vi "encryptSign.vi"(0 "HGF_GPG":refnum<class "HGF_GPG.lvclass">, 1 "options file":path, 2 "keyringfile":path, 3 "Sec keyringfile":path, 4 "string in":string, 5 "error in (no error)":errorcluster, 6 "key-id":string, 7 "reveicer array":string[](array[string]), 8 "receiver":string, 9 "password":string, 10 "Trust DB":path) -> (11 "success":bool=TRUE, 12 "dup Trust DB":path, 13 "data error":bool, 14 "dup HGF_GPG":refnum<class "HGF_GPG.lvclass">, 15 "dup options file":path, 16 "dup keyringfile":path, 17 "dup keyringfile 2":path, 18 "String out":string, 19 "error out":errorcluster)   [LabVIEW 2012, in "HGF_GPG.lvlib" / "HGF_GPG.lvclass"]
doc: "Encrypt a string. Only receiver in the list can decrypt the string."
uses:
  HGF_GPG.lvclass
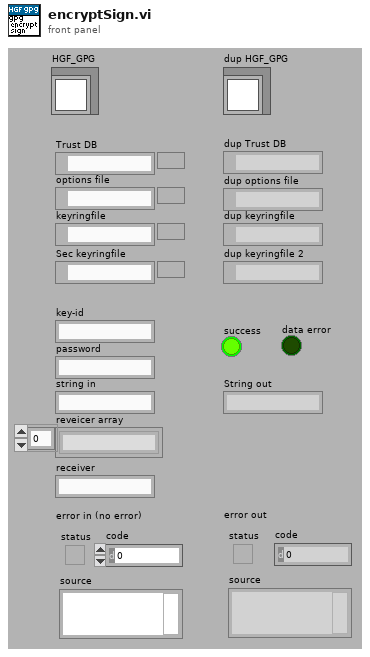
[diagram p1: front panel]
types:
  T1 = enum16{"open", "replace", "create", "open or create", "replace or create", "replace or create with confirmation"}
  T2 = enum16{"encrypt", "decrypt", "sign", "verify", "sign & encrypt", "verify & decrypt"}
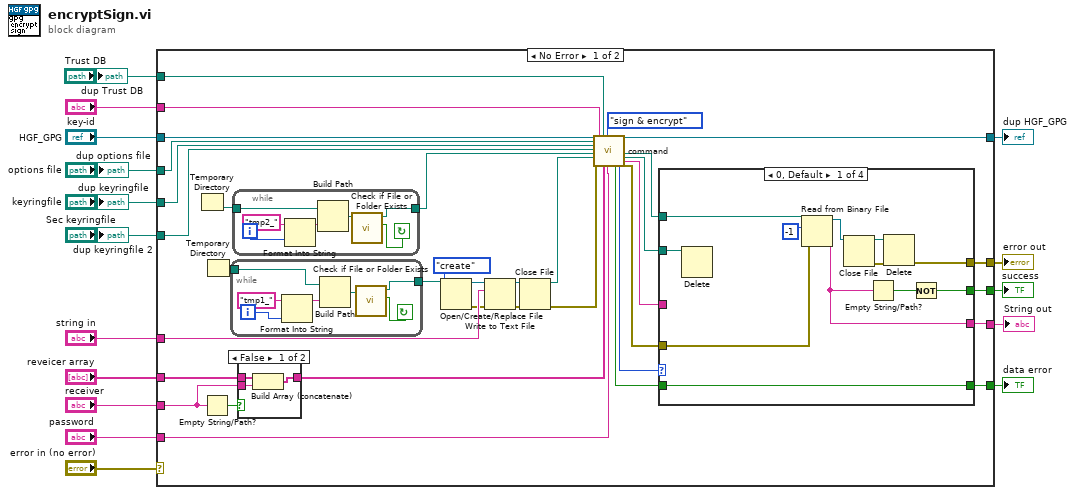
[diagram p0: block diagram]
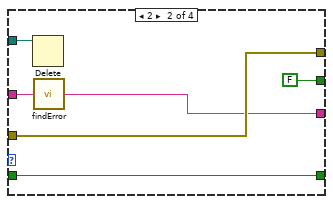
[diagram p3: hidden frame]
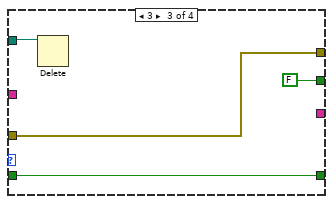
[diagram p4: hidden frame]
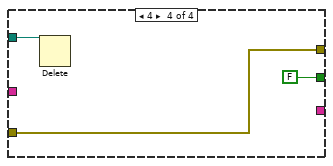
[diagram p5: hidden frame]
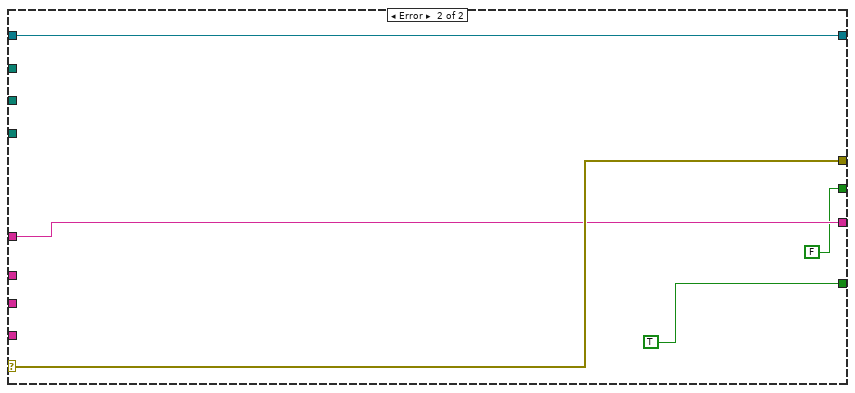
[diagram p6: hidden frame]
diagram:
  n1 = case shown="No Error" "error in (no error)" {
    selector: "error in (no error)" -> [_ w98]
    tunnel: [w50 w99] -> w14
    tunnel: "HGF_GPG" -> [w51 w99]
    tunnel: "receiver" -> [w32 _]
    tunnel: [w44 w98] -> w10
    tunnel: "string in" -> [w49 w97]
    tunnel: [w43 w97] -> w11
    tunnel: [w36 TRUE ("data error?")] -> w9
    tunnel: [w35 FALSE] -> w8
    tunnel: "reveicer array" -> [w34 _]
    tunnel: "password" -> [w25 _]
    tunnel: "key-id" -> [w19 _]
    tunnel: "keyringfile" -> [w29 _]
    tunnel: "options file" -> [w30 _]
    tunnel: "Sec keyringfile" -> [w18 _]
    tunnel: "Trust DB" -> [w17 _]
    frame No Error {
      n2 = Temporary Directory() -> (w38:path)
      n3 = Empty String/Path?(string/path=w32) -> (empty?=w33:bool)
      n4 = Temporary Directory() -> (w39:path)
      n5 = while {
        tunnel: [w94] -> w42
        tunnel: w39 -> [w92]
        i -> [w90]
        stop <- w93 continue-if-true
        n6 = Format Into String(initial string="tmp1_" ("name or relative path"), w90) -> (resulting string=w89:string)  [unwired: 2 in, 1 out]
        n7 = Build Path(base path=w92, name or relative path=w89) -> (appended path=w88:path)
        n8 = call <vilib>:"Check if File or Folder Exists.vi"("path"=w88) -> ("file or folder exists?"=w93:bool, "dup path"=w94:path)  [unwired: 1 in, 8 out]
      }
      n9 = while {
        tunnel: w38 -> [w87]
        tunnel: [w85] -> w28
        i -> [w83]
        stop <- w84 continue-if-true
        n10 = Format Into String(initial string="tmp2_" ("name or relative path"), w83) -> (resulting string=w82:string)  [unwired: 2 in, 1 out]
        n11 = Build Path(base path=w87, name or relative path=w82) -> (appended path=w86:path)
        n12 = call <vilib>:"Check if File or Folder Exists.vi"("path"=w86) -> ("file or folder exists?"=w84:bool, "dup path"=w85:path)  [unwired: 1 in, 8 out]
      }
      n13 = case shown="False" w33 {
        tunnel: [w54 w55] -> w26
        tunnel: w34 -> [w53 w55]
        tunnel: w32 -> [w52 _]
        frame False {
          n14 = Build Array (concatenate)(w53, w52) -> (w54:string[])
        }
        frame True {
        }
      }
      n15 = Open/Create/Replace File(file path (use dialog)=w42, operation (0:open)=T1."create") -> (refnum out=w41:refnum<file>, error out=w37:errorcluster)  [unwired: 1 in, 4 out]
      n16 = Write to Text File(file (use dialog)=w41, text=w49, error in=w37) -> (refnum out=w48:refnum<file>, error out=w47:errorcluster)  [unwired: 2 out]
      n17 = Close File(refnum=w48, error in=w47) -> (path=w27:path, error out=w46:errorcluster)
      n18 = call-dynamic "command.vi"("HGF_GPG"=w51, "options file"=w30, "keyringfile"=w29, "Sec keyringfile"=w18, "targetfile"=w28, "sourcefile"=w27, "error in (no error)"=w46, "key-id"=w19, "Trust DB"=w17, "reveiver"=w26, "task"=T2."sign & encrypt", "password"=w25) -> ("data error"=w45:bool, "return code"=w24:i32, "dup HGF_GPG"=w50:refnum<class "HGF_GPG.lvclass">, "dup targetfile"=w20:path, "dup sourcefile"=w21:path, "standard error"=w22:string, "error out"=w23:errorcluster)  [unwired: 1 in, 8 out]
      n19 = case shown="0, Default" w24 {
        tunnel: w22 -> [_ w72 _ _]
        tunnel: w23 -> [w58 w73 w77 w80]
        tunnel: w45 -> [w62 w69 w75 _]
        tunnel: [w65 w73 w77 w80] -> w44
        tunnel: [w61 w71 _ _] -> w43
        tunnel: [w62 w69 w75 _] -> w36
        tunnel: [w59 FALSE FALSE FALSE] -> w35
        tunnel: w21 -> [w57 w68 w74 w78]
        tunnel: w20 -> [w56 _ _ _]
        frame 0, Default {
          n20 = Delete(path (use dialog)=w57) -> ()  [unwired: 1 in, 6 out]
          n21 = Read from Binary File(8:w58, 10:-1 ("count (1)"), 11:w56) -> (2:w61:string, 3:w67:refnum<file>)  [unwired: 5 out]
          n22 = Close File(refnum=w67) -> (path=w64:path, error out=w66:errorcluster)  [unwired: 1 in]
          n23 = Empty String/Path?(string/path=w61) -> (empty?=w60:bool)
          n24 = Delete(path (use dialog)=w64, error in=w66) -> (error out=w65:errorcluster)  [unwired: 5 out]
          n25 = Not(x=w60) -> (.not. x?=w59:bool)
        }
        frame 2 {
          n26 = Delete(path (use dialog)=w68) -> ()  [unwired: 1 in, 6 out]
          n27 = call "findError.vi"("error string in"=w72) -> ("error out"=w71:string)
        }
        frame 3 {
          n28 = Delete(path (use dialog)=w74) -> ()  [unwired: 1 in, 6 out]
        }
        frame 4 {
          n29 = Delete(path (use dialog)=w78) -> ()  [unwired: 1 in, 6 out]
        }
      }
    }
    frame Error {
    }
  }
  "error out" <- w10
  "dup HGF_GPG" <- w14
  "String out" <- w11
  "success" <- w8
  "data error" <- w9
  "dup options file" <- "options file"
  "dup keyringfile" <- "keyringfile"
  "dup keyringfile 2" <- "Sec keyringfile"
  "dup Trust DB" <- "Trust DB"
